vi "Show and Hide Panel Controls.vi"(3 "VI Reference In":refnum<vi>, 4 "Operation":u16(ring) items=["Hide", "Show"], 5 "Items to Hide":string[](array[string])) -> (0 "VI Reference Out":refnum<vi>)   [LabVIEW 2016]
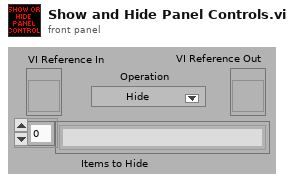
[diagram p1: front panel]
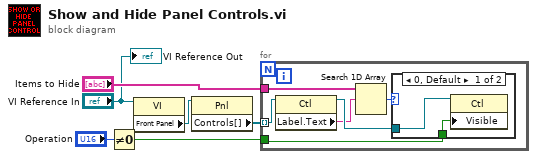
[diagram p0: block diagram]
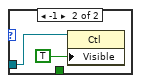
[diagram p2: hidden frame]
diagram:
  n1 = Not Equal To 0?(x="Operation") -> (x != 0?=w2:bool)
  n2 = property class="VI"(reference="VI Reference In") -> ("Front Panel"=w5:refnum<vi>)  [unwired: 1 in, 2 out]
  n3 = property class="Pnl"(reference=w5) -> ("Controls[]"=w4:refnum<vi>[])  [unwired: 1 in, 2 out]
  n4 = for {
    tunnel: "Items to Hide" -> [w10]
    tunnel: w4 -> [w12] mode=indexing
    tunnel: w2 -> [w7]
    n5 = property class="Ctl"(reference=w12) -> (reference out=w11:refnum<vi>, "Label.Text"=w9:string)  [unwired: 1 in, 1 out]
    n6 = Search 1D Array(1D array=w10, element=w9) -> (index of element=w8:i32)  [unwired: 1 in]
    n7 = case shown="0, Default" w8 {
      tunnel: w11 -> [w14 w16]
      tunnel: w7 -> [w13 _]
      frame 0, Default {
        n8 = property class="Ctl"(reference=w14, "Visible"=w13) -> ()  [unwired: 1 in, 2 out]
      }
      frame -1 {
        n9 = property class="Ctl"(reference=w16, "Visible"=TRUE) -> ()  [unwired: 1 in, 2 out]
      }
    }
  }
  "VI Reference Out" <- "VI Reference In"
